vi "cell simulator.vi"() -> ()   [LabVIEW 2017]
panel:
  in  "Tab Control":enum32{"PRINCIAPAL", "GRAPH 2"}(tab)
  out "Voc Graph":dbl[](graph)
  out "SOC graph":dbl[](graph)
  in  "capacity cell":dbl=10.0
  in  "temperature(ªC) battery not used":dbl
  in  "SOC_initial":dbl=100.0
  in  "Current":dbl=600.0
  in  "N cycles":dbl
  in  "Time cell\nnot used(months)":dbl
  in  "Cycling\ntemperature\nto K factors":u16(ring) items=["25ºC", "50ºC"]
  out "capacity usable(Ah)":dbl
  out "Rcycle":dbl
  in  "stop":bool
  out "XY Graph":cluster{"Waveform Graph":dbl[], dbl[]}(graph)
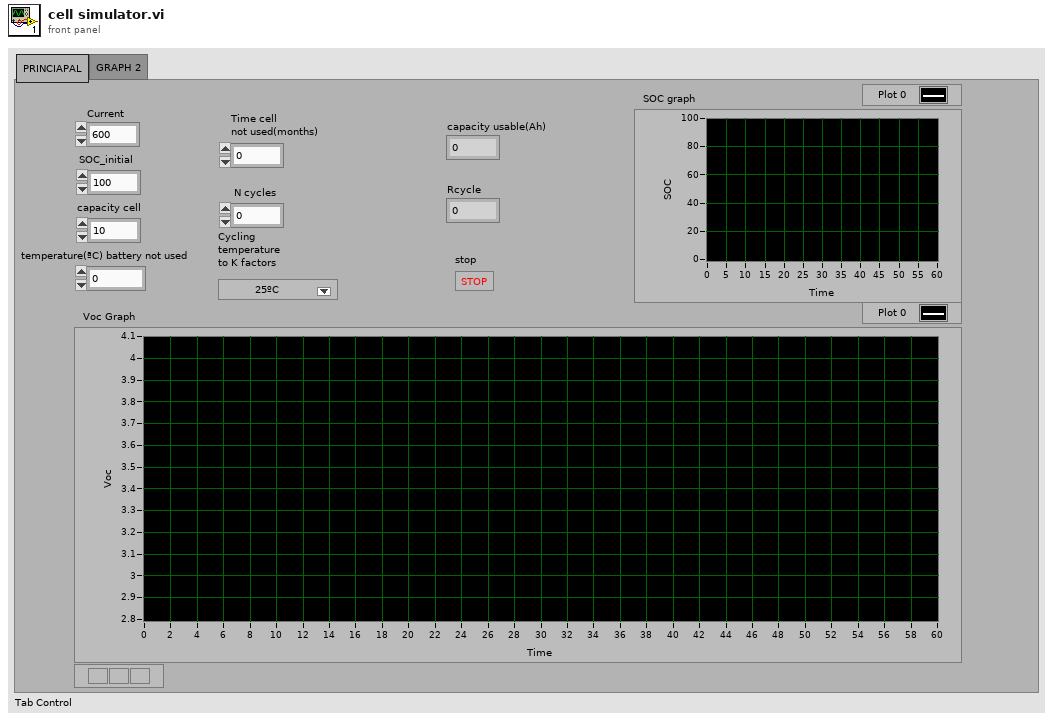
[diagram p1: front panel]
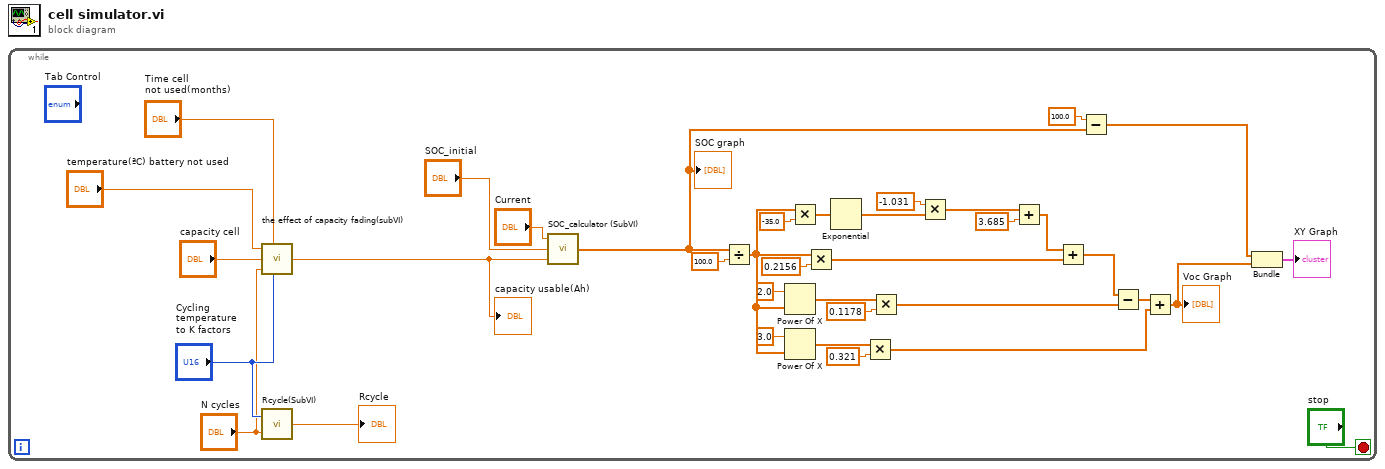
[diagram p0: block diagram]
diagram:
  n1 = while {
    stop <- "stop" stop-if-true
    n2 = call "the effect of capacity fading(subVI).vi"("temperature(ªC) battery not used"="temperature(ªC) battery not used", "Time cell\nnot used(months)"="Time cell\nnot used(months)", "capacity cell"="capacity cell", "N cycles"="N cycles", "Cycling\ntemperature\nto K factors"="Cycling\ntemperature\nto K factors") -> ("capacity \nusable"=w31:dbl)
    "capacity usable(Ah)" <- w31
    n3 = call "Rcycle(SubVI).vi"("N cycles"="N cycles", "Cycling\ntemperature\nto K factors"="Cycling\ntemperature\nto K factors") -> ("Rcycle"=→"Rcycle":dbl)
    n4 = call "SOC_calculator (SubVI).vi"("Capacity Usable"=w31, "SOC init"="SOC_initial", "Current"="Current") -> ("Waveform Graph"=w2:dbl[])
    "SOC graph" <- w2
    n5 = Divide(x=w2, y=100.0) -> (x/y=w6:dbl[])
    n6 = Power Of X(1:w6, 2:2.0 ("y")) -> (0:w15:dbl[])
    n7 = Power Of X(1:w6, 2:3.0 ("y")) -> (0:w10:dbl[])
    n8 = Multiply(x=w6, y=-35.0) -> (x*y=w25:dbl[])
    n9 = Multiply(x=w6, y=0.2156) -> (x*y=w19:dbl[])
    n10 = Exponential(1:w25) -> (0:w23:dbl[])
    n11 = Multiply(x=w10, y=0.321) -> (x*y=w9:dbl[])
    n12 = Multiply(x=w15, y=0.1178) -> (x*y=w14:dbl[])
    n13 = Multiply(x=-1.031, y=w23) -> (x*y=w21:dbl[])
    n14 = Add(x=w21, y=3.685) -> (x+y=w18:dbl[])
    n15 = Add(x=w18, y=w19) -> (x+y=w13:dbl[])
    n16 = Subtract(x=100.0, y=w2) -> (x-y=w1:dbl[])
    n17 = Subtract(x=w13, y=w14) -> (x-y=w8:dbl[])
    n18 = Add(x=w8, y=w9) -> (x+y=w5:dbl[])
    "Voc Graph" <- w5
    n19 = Bundle(w1, w5) -> (→"XY Graph":cluster{dbl[], dbl[]})  [unwired: 1 in]
  }
